vi "Measure.vi"(6 "Init work":bool, 7 "Update period":dbl, 8 "error in (no error)":errorcluster, 9 "Last request":bool, 10 "Requester":string, 11 "Lockin Digitizer in":refnum<class "Lockin Digitizer.lvclass">) -> (0 "error out":errorcluster, 3 "Lockin Digitizer out":refnum<class "Lockin Digitizer.lvclass">)   [LabVIEW 2021, in "Lockin Digitizer.lvclass"]
uses:
  Lockin Digitizer.lvclass
  C:/GitHub/LabActor/Template Module/Template Module.lvclass
  C:/Program Files/National Instruments/LabVIEW 2021/vi.lib/ActorFramework/Actor/Actor.lvclass
  Publish-Subscribe/Context.ctl
  Template Module/Template Module.lvclass/Template Module.ctl
  <vilib>/ActorFramework/Actor/Actor.lvclass/Actor.ctl
  NHMFL_Core/Libraries/Instruments/Results/Acquired Result/Acquired Result.lvclass/Acquired Result.ctl
  Publish-Subscribe/Interfaces/Subscriber Messages/Information Msg/Information Msg.lvclass/Information Msg.ctl
  <vilib>/ActorFramework/Message Enqueuer/Message Enqueuer.lvclass/Message Enqueuer.ctl
  Template Module/Read Name.vi
  NHMFL_Core/Libraries/Instruments/Results/Acquired Result/Write Sender.vi
  <vilib>/ActorFramework/Message Enqueuer/Enqueue.vi
  NHMFL_Core/Libraries/Instruments/Results/Acquired Result/Acquired Result.lvclass
  C:/GitHub/LabActor/Publish-Subscribe/Interfaces/Information/Information.lvclass
  Publish-Subscribe/Interfaces/Subscriber Messages/Information Msg/Information Msg.lvclass
  C:/Program Files/National Instruments/LabVIEW 2021/vi.lib/ActorFramework/Message/Message.lvclass
  <vilib>/ActorFramework/Message Priority Queue/Priority Enqueue.vi
  NHMFL_Core/Libraries/Instruments/Pulse Driver/Lockin Digitizer Driver/Lockin Digitizer Driver.lvclass
  Lockin Digitizer.lvclass/Lockin Digitizer.ctl
  <vilib>/ActorFramework/Actor/Actor.lvclass
  C:/GitHub/LabActor/Pulse Recorders/Pulse Recorder Actor/Pulse Recorder Actor.lvclass
  C:/GitHub/LabActor/Instrument Actor/Instrument Actor.lvclass
  C:/GitHub/LabActor/Worker/Worker Actor/Worker Actor.lvclass
  C:/GitHub/LabActor/Worker/Woker Interface/Worker.lvclass
  C:/GitHub/LabActor/Pulse Recorders/Interfaces/Pulse Recorder/Pulse Recorder.lvclass
  C:/GitHub/LabActor/Pulse Recorders/Lockin Digitizer/Lockin Digitizer.lvclass
  C:/GitHub/LabActor/Recorders/Interfaces/Continuous Recorder/Continuous Recorder.lvclass
  C:/GitHub/NHMFL_Core/Libraries/Instruments/Results/Acquired Result/Acquired Result.lvclass
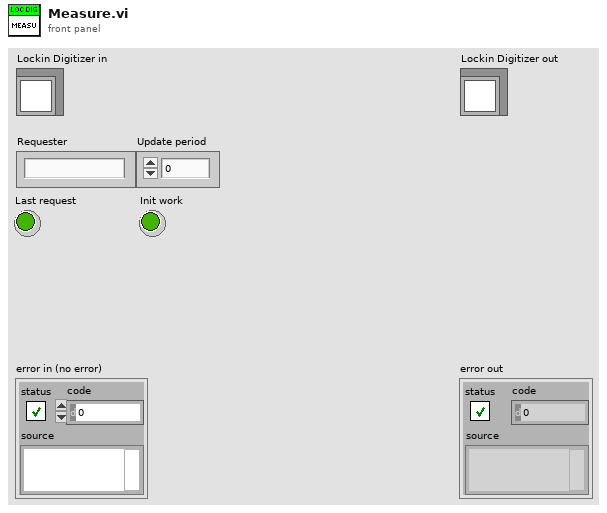
[diagram p1: front panel]
types:
  T1 = typedef "Context.ctl" = cluster{"Topic":string, "Source":string}
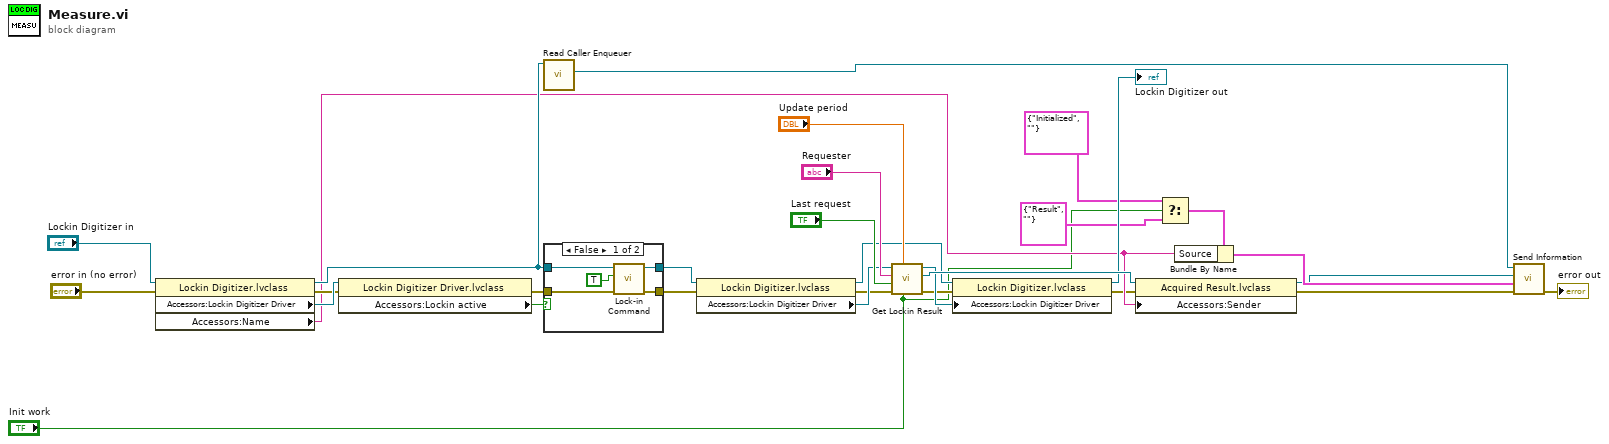
[diagram p0: block diagram]
diagram:
  n1 = property class="Lockin Digitizer.lvclass"(reference="Lockin Digitizer in", error in="error in (no error)") -> (reference out=w16:refnum<class "Lockin Digitizer.lvclass">, error out=w18:errorcluster, "Accessors:Lockin Digitizer Driver"=w19:refnum<class "Lockin Digitizer Driver.lvclass">, "Accessors:Name"=w8:string)
  n2 = property class="Lockin Digitizer Driver.lvclass"(reference=w19, error in=w18) -> (error out=w15:errorcluster, "Accessors:Lockin active"=w17:bool)  [unwired: 1 out]
  n3 = call <vilib>:"Read Caller Enqueuer.vi"("Actor"=w16) -> ("Caller Enqueuer"=w6:refnum<class "Message Enqueuer.lvclass">)  [unwired: 10 in]
  n4 = case shown="False" w17 {
    tunnel: w16 -> [w35 w37]
    tunnel: w15 -> [w33 w36]
    tunnel: [w32 w37] -> w14
    tunnel: [w31 w36] -> w13
    frame False {
      n5 = call-dynamic "Lock-in Command.vi"("error in (no error)"=w33, "Lock-in"=TRUE, "Lockin Digitizer in"=w35) -> ("error out"=w31:errorcluster, "Lockin Digitizer out"=w32:refnum<class "Lockin Digitizer.lvclass">)  [unwired: 6 in, 1 out]
    }
    frame True {
    }
  }
  n6 = property class="Lockin Digitizer.lvclass"(reference=w14, error in=w13) -> (reference out=w10:refnum<class "Lockin Digitizer.lvclass">, error out=w11:errorcluster, "Accessors:Lockin Digitizer Driver"=w12:refnum<class "Lockin Digitizer Driver.lvclass">)
  n7 = call-dynamic "Get Lockin Result.vi"("Init work"="Init work", "Update period"="Update period", "error in (no error)"=w11, "Last request"="Last request", "Requester"="Requester", "Lockin Digitizer Driver in"=w12) -> ("error out"=w24:errorcluster, "Result out"=w27:refnum<class "Acquired Result.lvclass">, "Lockin Digitizer Driver out"=w26:refnum<class "Lockin Digitizer Driver.lvclass">)  [unwired: 2 in, 1 out]
  n8 = property class="Lockin Digitizer.lvclass"(reference=w10, error in=w24, "Accessors:Lockin Digitizer Driver"=w26) -> (reference out=→"Lockin Digitizer out":refnum<class "Lockin Digitizer.lvclass">, error out=w7:errorcluster)
  n9 = property class="Acquired Result.lvclass"(reference=w27, error in=w7, "Accessors:Sender"=w8) -> (reference out=w9:refnum<class "Acquired Result.lvclass">, error out=w5:errorcluster)
  n10 = Select(t=T1 {"Topic"="Initialized", "Source"=""} ("Context"), s="Init work", f=T1 {"Topic"="Result", "Source"=""} ("Context")) -> (s? t:f=w3:T1)
  n11 = Bundle By Name(cluster=w3, "Source"=w8) -> (w28:T1)
  n12 = call "Send Information.vi"("error in (no error)"=w5, "Context"=w28, "Information"=w9, "Message Enqueuer"=w6) -> ("error out"=→"error out":errorcluster)  [unwired: 6 in, 1 out]
